vi "Write Port.vi"(8 "error in (no error)":errorcluster, 10 "Port":u16, 11 "TcpSocket in":refnum<class "TcpSocket.lvclass">) -> (0 "error out":errorcluster, 3 "TcpSocket out":refnum<class "TcpSocket.lvclass">)   [LabVIEW 2021, in "TcpSocket.lvlib" / "TcpSocket.lvclass"]
uses:
  TcpSocket.lvclass
  TcpSocket.lvclass/TcpSocket.ctl
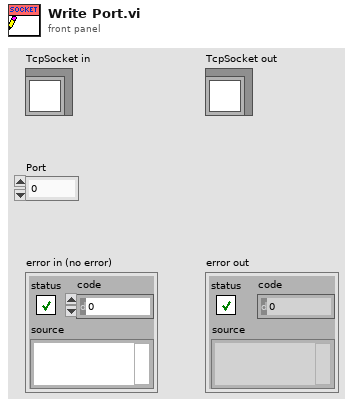
[diagram p1: front panel]
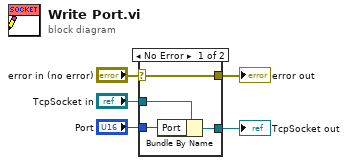
[diagram p0: block diagram]
diagram:
  n1 = case shown="No Error" "error in (no error)" {
    selector: "error in (no error)" -> [w9 w10]
    tunnel: [w9 w10] -> w4
    tunnel: [w7 w11] -> w2
    tunnel: "TcpSocket in" -> [w8 w11]
    tunnel: "Port" -> [w6 _]
    frame No Error {
      n2 = Bundle By Name(cluster=w8, "Port"=w6) -> (w7:refnum<class "TcpSocket.lvclass">)
    }
    frame Error {
    }
  }
  "error out" <- w4
  "TcpSocket out" <- w2
